vi "AWG Initialize.vi"(8 "error in (no error)":errorcluster, 9 "Reset (True)":bool=TRUE, 10 "ID Query (True)":bool=TRUE, 11 "awg session in":T1) -> (0 "error out":errorcluster, 2 "idn string":string, 3 "awg session out":T1)   [LabVIEW 2013, in "AWG.lvlib"]
doc: "AWG wrapper: initialize function generator."
uses:
  AWG.lvlib
  AWG Session.ctl
  AWG Type.ctl
  Agilent 33XXX Series/Agilent 33XXX Series.lvlib
  Agilent 3352X Series/Agilent 3352X Series.lvlib
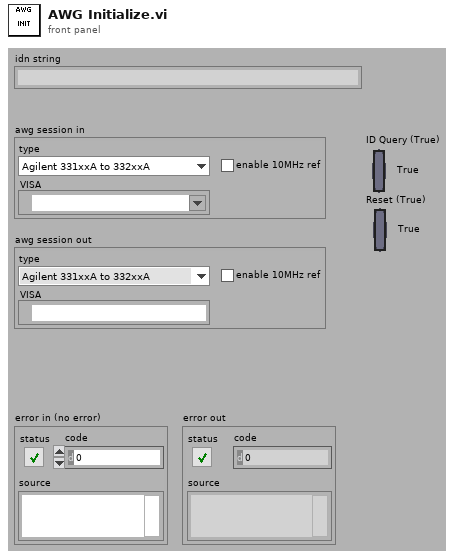
[diagram p1: front panel]
types:
  T1 = typedef "AWG.lvlib/AWG Session.ctl" = cluster{"type":T2, "VISA":refnum<visa-resource-name>, "enable 10MHz ref":bool}
  T2 = typedef "AWG.lvlib/AWG Type.ctl" = enum16{"Agilent 331xxA to 332xxA", "Agilent 335xxA to 336xxA", "dummy"}
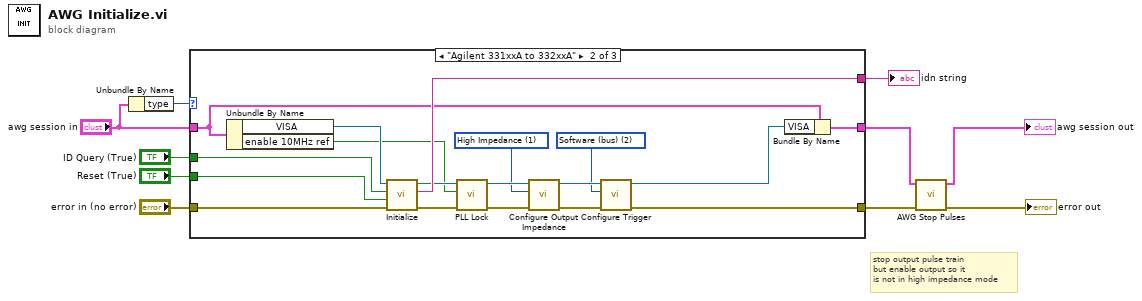
[diagram p0: block diagram]
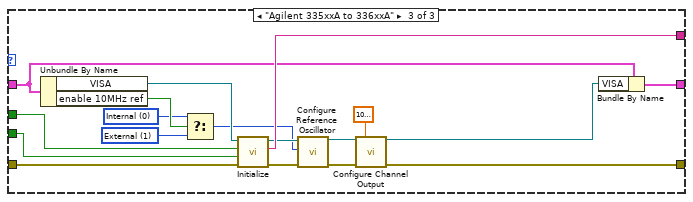
[diagram p3: hidden frame]
diagram:
  # "stop output pulse train\nbut enable output so it \nis not in high impedance mode"
  n1 = Unbundle By Name("awg session in") -> ("type"=w10:T2)
  n2 = case shown="\"Agilent 331xxA to 332xxA\"" w10 {
    tunnel: "error in (no error)" -> [w12 w30 w48]
    tunnel: [_ w29 w47] -> w8
    tunnel: [w12 w13 w32] -> w4
    tunnel: "awg session in" -> [w11 w26 w45]
    tunnel: [w11 w27 w44] -> w2
    tunnel: "ID Query (True)" -> [_ w25 w39]
    tunnel: "Reset (True)" -> [_ w24 w38]
    frame Default {
    }
    frame "Agilent 331xxA to 332xxA" {
      w15 = u16 2 items=["Internal", "External", "Software (bus)"] ("Trigger Source (0: Internal)")
      w18 = u16 1 items=["50 Ohms", "High Impedance", "User Defined"] ("Impedance (0: 50 Ohms)")
      n3 = Unbundle By Name(w26) -> ("VISA"=w28:refnum<visa-resource-name>, "enable 10MHz ref"=w21:bool)
      n4 = call "Initialize.vi"("error in (no error)"=w30, "Reset (True)"=w24, "ID Query (True)"=w25, "VISA resource name"=w28) -> ("error out"=w23:errorcluster, "idn string"=w29:string, "VISA resource name out"=w22:refnum<visa-resource-name>)  [unwired: 5 in]
      n5 = call "PLL Lock.vi"("error in (no error)"=w23, "PLL lock  (T: Enable)"=w21, "VISA resource name"=w22) -> ("error out"=w20:errorcluster, "VISA resource name out"=w19:refnum<visa-resource-name>)  [unwired: 7 in]
      n6 = call "Configure Output Impedance.vi"("error in (no error)"=w20, "Impedance (0: 50 Ohms)"=w18, "VISA resource name"=w19) -> ("error out"=w17:errorcluster, "VISA resource name out"=w16:refnum<visa-resource-name>)  [unwired: 7 in]
      n7 = call "Configure Trigger.vi"("error in (no error)"=w17, "Trigger Source (0: Internal)"=w15, "VISA resource name"=w16) -> ("error out"=w13:errorcluster, "VISA resource name out"=w14:refnum<visa-resource-name>)  [unwired: 7 in]
      n8 = Bundle By Name(cluster=w26, "VISA"=w14) -> (w27:T1)
    }
    frame "Agilent 335xxA to 336xxA" {
      w36 = 1 items=["Internal", "External"] ("Source (0: Internal)")
      w37 = 0 items=["Internal", "External"] ("Source (0: Internal)")
      n9 = Unbundle By Name(w45) -> ("VISA"=w46:refnum<visa-resource-name>, "enable 10MHz ref"=w41:bool)
      n10 = Select(t=w37, s=w41, f=w36) -> (s? t:f=w40:i32)
      n11 = call "Initialize.vi"("error in (no error)"=w48, "Reset (Enable)"=w38, "ID Query (Enable)"=w39, "VISA resource name"=w46) -> ("error out"=w42:errorcluster, "idn string"=w47:string, "VISA resource name out"=w43:refnum<visa-resource-name>)  [unwired: 5 in]
      n12 = call "Configure Reference Oscillator.vi"("error in (no error)"=w42, "Source (0: Internal)"=w40, "VISA resource name"=w43) -> ("error out"=w35:errorcluster, "VISA resource name out"=w34:refnum<visa-resource-name>)  [unwired: 7 in]
      n13 = call "Configure Channel Output.vi"("VISA resource name"=w34, "Output Impedance (50 Ohm)"=1000000.0, "error in (no error)"=w35) -> ("VISA resource name out"=w33:refnum<visa-resource-name>, "error out"=w32:errorcluster)  [unwired: 11 in]
      n14 = Bundle By Name(cluster=w45, "VISA"=w33) -> (w44:T1)
    }
  }
  "idn string" <- w8
  n15 = call "AWG Stop Pulses.vi"("error in (no error)"=w4, "awg session in"=w2) -> ("error out"=→"error out":errorcluster, "awg session out"=→"awg session out":T1)  [unwired: 8 in]
